vi "显示图片.vi"() -> ()   [LabVIEW 2018]
uses:
  <vilib>/picture/picture.llb/Draw True-Color Pixmap.vi
panel:
  out "二维图片":picture
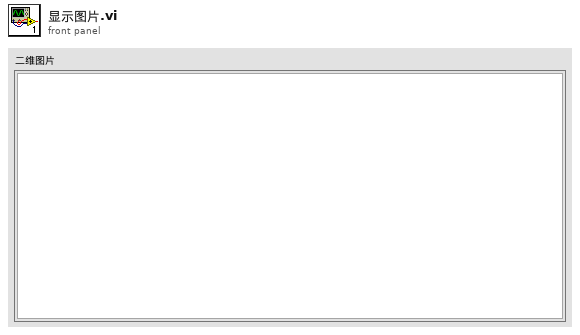
[diagram p1: front panel]
types:
  T1 = typedef "imagedata.ctl" = cluster{"image type":i32, "image depth":i32, "image":u8[], "mask":u8[], "colors":u32[], "Rectangle":cluster{"left":i16, "top":i16, "right":i16, "bottom":i16}}
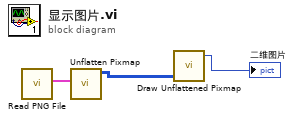
[diagram p0: block diagram]
diagram:
  n1 = call <vilib>:"Read PNG File.vi"() -> ("image data"=w1:T1)  [unwired: 9 in, 2 out]
  n2 = call <vilib>:"Unflatten Pixmap.vi"("image data"=w1) -> ("24-bit pixmap"=w2:u32[][])  [unwired: 4 in, 6 out]
  n3 = call-poly <vilib>:"Draw Unflattened Pixmap.vi"("data (RGB format)"=w2) -> ("new picture"=→"二维图片":picture)  [unwired: 8 in]
